vi "Add Process.vi"(8 "error in (no error)":errorcluster, 10 "Process":refnum<class "Process.lvclass">, 11 "Rig In":refnum<class "Application.lvclass">) -> (0 "error out":errorcluster, 3 "Rig Out":refnum<class "Application.lvclass">)   [LabVIEW 2020, in "Application.lvclass"]
doc: "Add a process to the application. The process should be initialized before being added to the application. After adding a proess, the lifecycle of the process is owned and managed by the owining application. It is therefore not necessary to Start, Stop, or Clear added processes."
uses:
  Application.lvclass
  C:/Users/AntonSundqvist/Documents/GitHub/Triarc-Framework/source/Framework/Process/Process.lvclass
  Process/Process.lvclass
  Process/Public/Lifecycle/Lifecycle State.ctl
  Process/Process.lvclass/Process.ctl
  Application.lvclass/Application.ctl
  <vilib>/AdvancedString/1D String Array to Delimited String.vi
  <vilib>/Utility/error.llb/Clear Errors.vi
  <vilib>/Utility/error.llb/Error Cluster From Error Code.vi
  <vilib>/ErrorRing/Error Ring.xnode
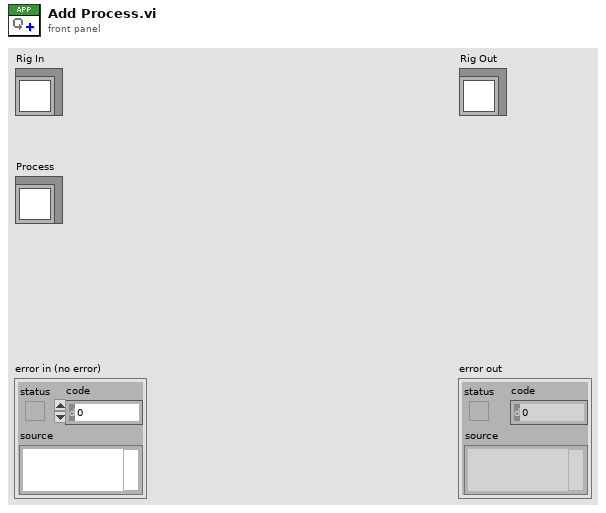
[diagram p1: front panel]
types:
  T1 = typedef "Process.lvclass/Lifecycle State.ctl" = enum16{"Uninitialized", "Initialized", "Started", "Running", "Stopped", "Finished"}
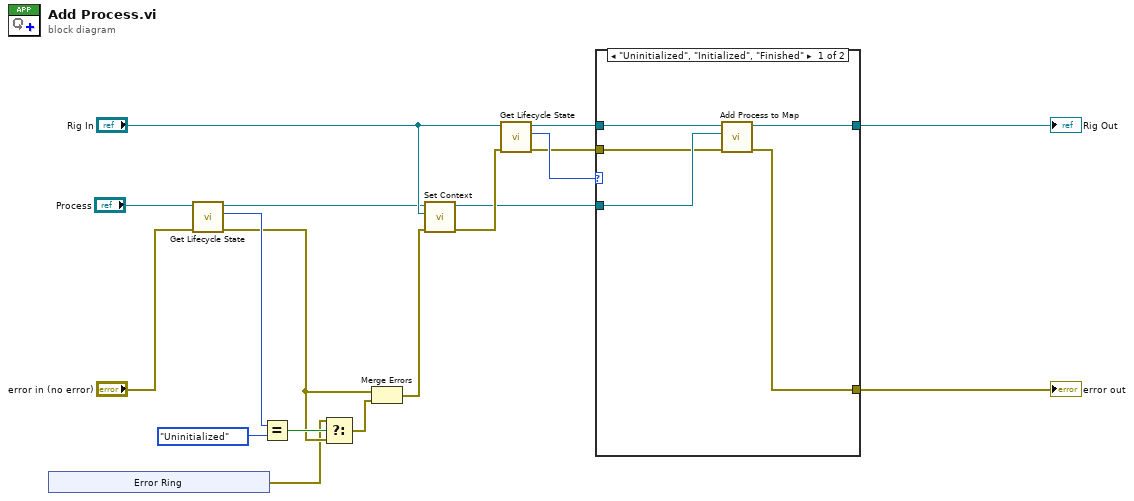
[diagram p0: block diagram]
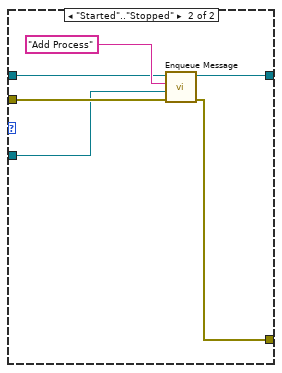
[diagram p2: hidden frame]
diagram:
  n1 = xnode "Error Ring"() -> ("error out"=w5:errorcluster)
  n2 = call "Get Lifecycle State.vi"("error in (no error)"="error in (no error)", "Process In"="Process") -> ("error out"=w7:errorcluster, "Lifecycle State"=w9:T1, "Process Out"=w3:refnum<class "Process.lvclass">)  [unwired: 6 in, 1 out]
  n3 = Equal?(x=w9, y=Lifecycle_State."Uninitialized" ("Lifecycle State")) -> (x = y?=w8:bool)
  n4 = Select(t=w5, s=w8, f=w7) -> (s? t:f=w6:errorcluster)
  n5 = Merge Errors(w7, w6) -> (w2:errorcluster)
  n6 = call "Set Context.vi"("error in (no error)"=w2, "Process Context"="Rig In", "Process In"=w3) -> ("error out"=w15:errorcluster, "Process Out"=w12:refnum<class "Process.lvclass">)  [unwired: 7 in]
  n7 = call "Get Lifecycle State.vi"("error in (no error)"=w15, "Process In"="Rig In") -> ("error out"=w11:errorcluster, "Lifecycle State"=w14:T1, "Process Out"=w13:refnum<class "Application.lvclass">)  [unwired: 6 in, 1 out]
  n8 = case shown="\"Uninitialized\", \"Initialized\", \"Finished\"" w14 {
    tunnel: [w23 w28] -> w18
    tunnel: [w20 w26] -> w17
    tunnel: w12 -> [w21 w24]
    tunnel: w13 -> [w22 w27]
    tunnel: w11 -> [w19 w25]
    frame "Uninitialized", "Initialized", "Finished" {
      n9 = call "Add Process to Map.vi"("error in (no error)"=w19, "Process Out"=w21, "Application in"=w22) -> ("error out"=w20:errorcluster, "Application out"=w23:refnum<class "Application.lvclass">)  [unwired: 7 in]
    }
    frame "Started".."Stopped" {
      n10 = call "Enqueue Message.vi"("error in (no error)"=w25, "Message Data"=w24, "Message"="Add Process", "Process In"=w27) -> ("error out"=w26:errorcluster, "Process Out"=w28:refnum<class "Application.lvclass">)  [unwired: 6 in]
    }
  }
  "error out" <- w17
  "Rig Out" <- w18
